vi "formulaNode.vi"() -> ()   [LabVIEW 2014]
panel:
  out "Conditional Function":cluster{"yValues":dbl[], "xValues":dbl[]}(graph)
  out "Sum Of Y Values":dbl(knob) scale=0.0..200.0
  in  "Step Size":dbl(knob)=3.0 scale=0.0..10.0
  in  "Frequency":dbl(knob)=0.3 scale=0.0..1.0
  in  "Amplitude":dbl(knob)=3.0 scale=0.0..10.0
  in  "Number of Elements":i32(knob)=50 scale=0.0..100.0
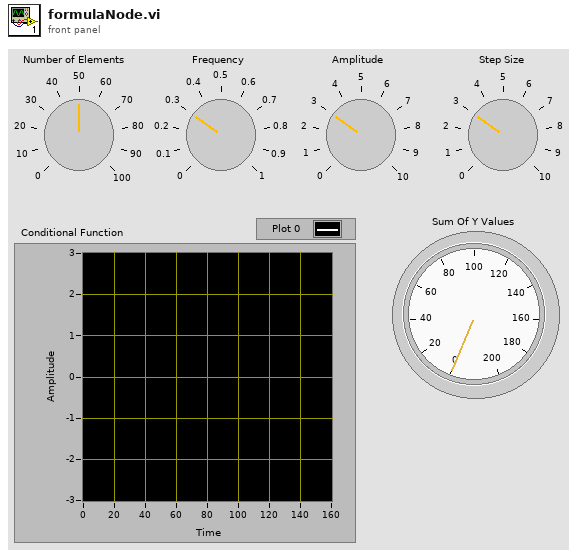
[diagram p1: front panel]
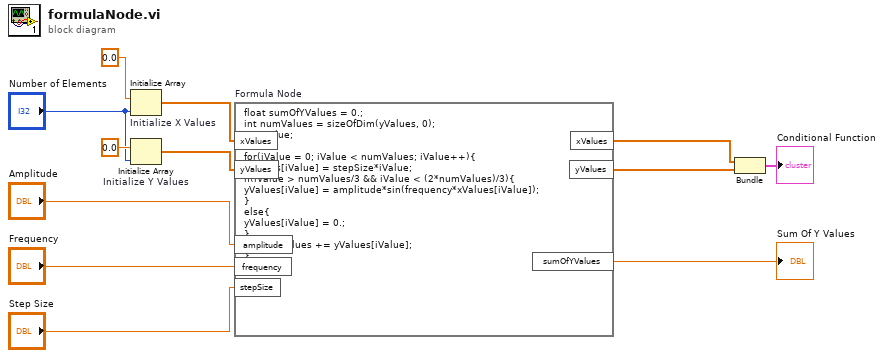
[diagram p0: block diagram]
diagram:
  n1 = Initialize Array "Initialize X Values"(0.0 ("element"), "Number of Elements") -> (w8:dbl[])
  n2 = Initialize Array "Initialize Y Values"(0.0 ("element"), "Number of Elements") -> (w9:dbl[])
  n3 = formula code="float sumOfYValues = 0.;\nint numValues = sizeOfDim(yValues, 0);\nint iValue;\n\nfor(iValue = 0; iValue < numValues; iValue++){\nxValues[iValue] = stepSize*iValue;\nif(iValue > numValues/3 && iValue < (2*numValues)/3){\nyValues[iValue] = amplitude*sin(frequency*xValues[iValue]);\n} \nelse{\nyValues[iValue] = 0.;\n}\nsumOfYValues += yValues[iValue];\n}"("yValues"=w9, "xValues"=w8, "amplitude"="Amplitude", "frequency"="Frequency", "stepSize"="Step Size") -> ("yValues"=w2:dbl[], "xValues"=w1:dbl[], "sumOfYValues"=→"Sum Of Y Values":dbl)
  n4 = Bundle("xValues"=w1, "yValues"=w2) -> (→"Conditional Function":cluster{"xValues":dbl[], "yValues":dbl[]})  [unwired: 1 in]
